vi "optagefrekvenssignal0.2.vi"() -> ()   [LabVIEW 2014]
uses:
  <vilib>/measure/maspectr.llb/FFT Power Spectrum and PSD for 1 Chan.vi
  <vilib>/measure/NI_MAPro.lvlib
panel:
  out "Max frequency":dbl
  out "FFT power spectre":cluster{"f0":dbl, "df":dbl, "magnitude":dbl[]}(graph)
  out "Soundsignal":waveform(dbl)(graph)
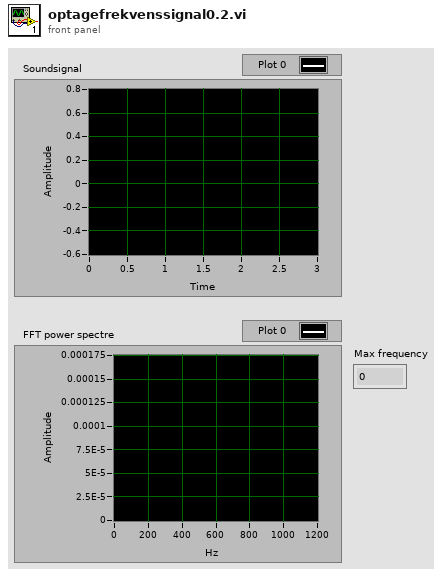
[diagram p1: front panel]
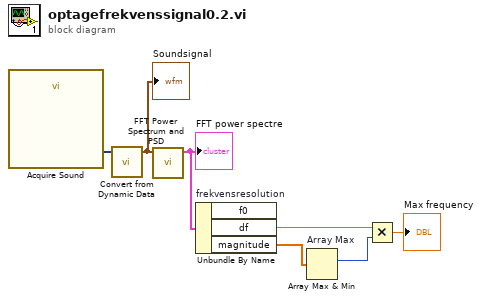
[diagram p0: block diagram]
diagram:
  n1 = call "Acquire Sound"() -> ("Data"=w3:dynamicdata)  [unwired: 18 in, 1 out]
  n2 = call "Convert from Dynamic Data"("Dynamic Data Type"=w3) -> ("Waveform"=w7:waveform(dbl))  [unwired: 3 in]
  "Soundsignal" <- w7
  n3 = call-poly <vilib>:"FFT Power Spectrum and PSD.vi"("time signal"=w7) -> ("Power Spectrum / PSD"=w6:cluster{"f0":dbl, "df":dbl, "magnitude":dbl[]})  [unwired: 7 in, 3 out]
  "FFT power spectre" <- w6
  n4 = Unbundle By Name "frekvensresolution"(w6) -> ("df"=w4:dbl, "magnitude"=w5:dbl[])  [unwired: 1 out]
  n5 = Array Max & Min "Array Max"(array=w5) -> (max index (indices)=w1:i32)  [unwired: 3 out]
  n6 = Multiply(x=w4, y=w1) -> (x*y=→"Max frequency":dbl)
